vi "Trilateration.vi"(8 "direction":bool, 9 "Point 3":cluster{"x":dbl, "y":dbl, "z":dbl, "r":dbl}={"x"=0.0, "y"=0.0, "z"=0.5, "r"=1.0}, 10 "Point 2":cluster{"x":dbl, "y":dbl, "z":dbl, "r":dbl}={"x"=0.0, "y"=1.0, "z"=1.0, "r"=1.0}, 11 "Point 1":cluster{"x":dbl, "y":dbl, "z":dbl, "r":dbl}={"x"=1.0, "y"=0.0, "z"=0.0, "r"=1.0}) -> (1 "new point z":dbl=0.11811869208701314, 2 "new point y":dbl=0.8159406539564933, 3 "new point x":dbl=0.4340593460435067)   [LabVIEW 2015]
doc: "Calculates position of a point in 3D space which is at known distances from three points."
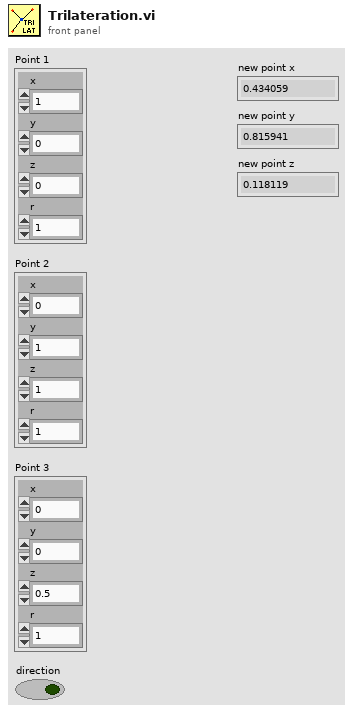
[diagram p1: front panel]
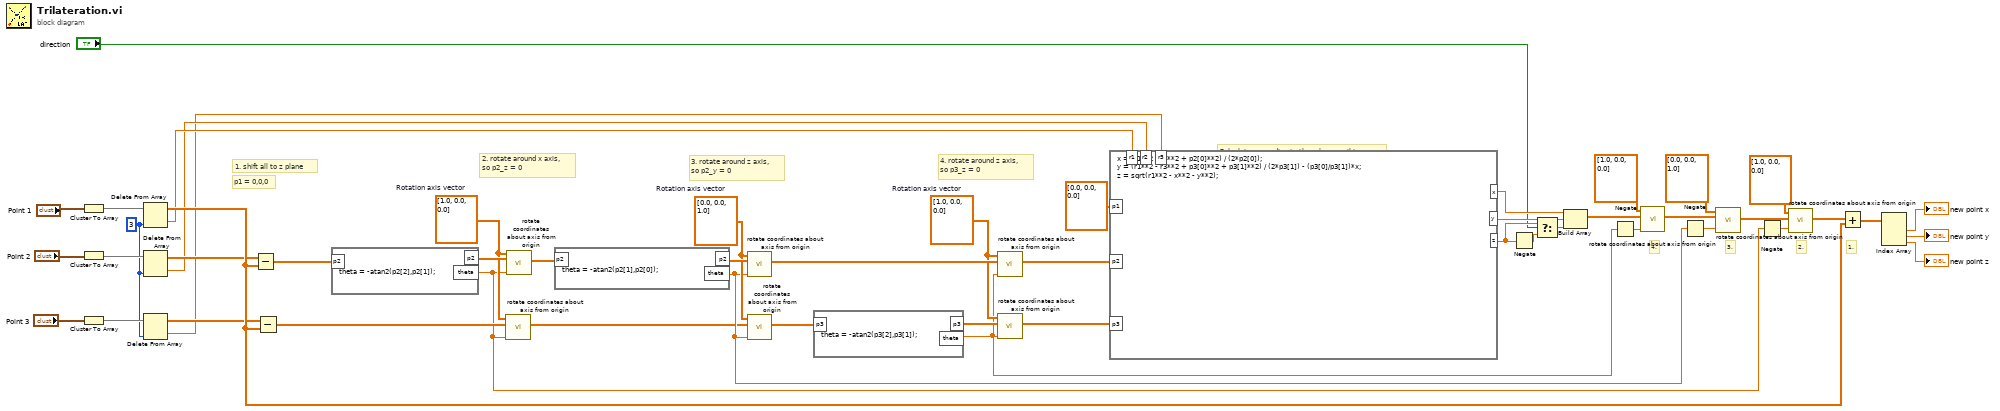
[diagram p0: block diagram]
diagram:
  w12 = 3 ("index")
  w30 = dbl[] [1.0, 0.0, 0.0]  # Rotation axis vector
  w38 = dbl[] [1.0, 0.0, 0.0]  # Rotation axis vector
  w50 = dbl[] [0.0, 0.0, 1.0]  # Rotation axis vector
  # "1."
  # "2."
  # "3."
  # "4."
  # "Calculate, according to the rules on wiki"
  # "4. rotate around z axis,\nso p3_z = 0"
  # "2. rotate around x axis,\nso p2_z = 0"
  # "1. shift all to z plane"
  # "3. rotate around z axis,\nso p2_y = 0"
  # "p1 = 0,0,0"
  n1 = Cluster To Array(cluster="Point 1") -> (array=w13:dbl[])
  n2 = Cluster To Array(cluster="Point 2") -> (array=w14:dbl[])
  n3 = Cluster To Array(cluster="Point 3") -> (array=w17:dbl[])
  n4 = Delete From Array(array=w13, index=w12) -> (deleted portion=w8:dbl, array with subset deleted=w11:dbl[])  [unwired: 1 in]
  n5 = Delete From Array(array=w14, index=w12) -> (deleted portion=w7:dbl, array with subset deleted=w10:dbl[])  [unwired: 1 in]
  n6 = Delete From Array(array=w17, index=w12) -> (deleted portion=w6:dbl, array with subset deleted=w9:dbl[])  [unwired: 1 in]
  n7 = Subtract(x=w10, y=w11) -> (x-y=w40:dbl[])
  n8 = Subtract(x=w9, y=w11) -> (x-y=w39:dbl[])
  n9 = formula code="theta = -atan2(p2[2],p2[1]);"("p2"=w40) -> ("theta"=w28:dbl, "p2"=w41:dbl[])
  n10 = call "rotate coordinates about axis from origin.vi"("Angle (CCW)"=w28, "Point to rotate"=w39, "Rotation axis vector"=w38) -> ("New position"=w36:dbl[])  [unwired: 8 in]
  n11 = call "rotate coordinates about axis from origin.vi"("Angle (CCW)"=w28, "Point to rotate"=w41, "Rotation axis vector"=w38) -> ("New position"=w37:dbl[])  [unwired: 8 in]
  n12 = formula code="theta = -atan2(p2[1],p2[0]);"("p2"=w37) -> ("theta"=w45:dbl, "p2"=w51:dbl[])
  n13 = call "rotate coordinates about axis from origin.vi"("Angle (CCW)"=w45, "Point to rotate"=w51, "Rotation axis vector"=w50) -> ("New position"=w32:dbl[])  [unwired: 8 in]
  n14 = call "rotate coordinates about axis from origin.vi"("Angle (CCW)"=w45, "Point to rotate"=w36, "Rotation axis vector"=w50) -> ("New position"=w35:dbl[])  [unwired: 8 in]
  n15 = formula code="theta = -atan2(p3[2],p3[1]);"("p3"=w35) -> ("theta"=w24:dbl, "p3"=w34:dbl[])
  n16 = call "rotate coordinates about axis from origin.vi"("Angle (CCW)"=w24, "Point to rotate"=w32, "Rotation axis vector"=w30) -> ("New position"=w31:dbl[])  [unwired: 8 in]
  n17 = call "rotate coordinates about axis from origin.vi"("Angle (CCW)"=w24, "Point to rotate"=w34, "Rotation axis vector"=w30) -> ("New position"=w33:dbl[])  [unwired: 8 in]
  n18 = formula code="x = (r1**2 - r2**2 + p2[0]**2) / (2*p2[0]);\ny = (r1**2 - r3**2 + p3[0]**2 + p3[1]**2) / (2*p3[1]) - (p3[0]/p3[1])*x;\nz = sqrt(r1**2 - x**2 - y**2);"("p1"=dbl[] [0.0, 0.0, 0.0] ("input variable"), "p2"=w31, "p3"=w33, "r1"=w8, "r2"=w7, "r3"=w6) -> ("x"=w48:dbl, "y"=w47:dbl, "z"=w43:dbl)
  n19 = Negate(x=w43) -> (-x=w44:dbl)
  n20 = Select(t=w43, s="direction", f=w44) -> (s? t:f=w42:dbl)
  n21 = Build Array(w48, w47, w42) -> (w26:dbl[])
  n22 = Negate(x=w24) -> (-x=w27:dbl)
  n23 = call "rotate coordinates about axis from origin.vi"("Angle (CCW)"=w27, "Point to rotate"=w26, "Rotation axis vector"=dbl[] [1.0, 0.0, 0.0]) -> ("New position"=w23:dbl[])  [unwired: 8 in]
  n24 = Negate(x=w45) -> (-x=w29:dbl)
  n25 = call "rotate coordinates about axis from origin.vi"("Angle (CCW)"=w29, "Point to rotate"=w23, "Rotation axis vector"=dbl[] [0.0, 0.0, 1.0]) -> ("New position"=w20:dbl[])  [unwired: 8 in]
  n26 = Negate(x=w28) -> (-x=w21:dbl)
  n27 = call "rotate coordinates about axis from origin.vi"("Angle (CCW)"=w21, "Point to rotate"=w20, "Rotation axis vector"=dbl[] [1.0, 0.0, 0.0]) -> ("New position"=w19:dbl[])  [unwired: 8 in]
  n28 = Add(x=w19, y=w11) -> (x+y=w4:dbl[])
  n29 = Index Array(array=w4) -> (element #1=→"new point x":dbl, element #2=→"new point y":dbl, element #3=→"new point z":dbl)  [unwired: 3 in]
